vi "Basic Set Address.vi"(6 "chip select  (1st chip)":enum16{"1st chip", "2nd chip"}(ring), 7 "address type (DDRAM)":enum16{"DDRAM", "CGRAM"}(ring), 8 "error in (no error)":errorcluster, 9 "address (0, 0)":u8 format="%.0x", 11 "cluster of private data in":T1={"FPGA VI Reference"=refnum, "device index"=0, "screen size"=enum."8x1", "font size"=enum."5x8", "auto wrap"=FALSE, "alignment"=enum."None", "number of line"=enum."2 lines", "shift 0"=0, "entry mode 0"=enum."increment & no shift", "shift 1"=0, "entry mode 1"=enum."increment & no shift"}) -> (0 "error out":errorcluster, 3 "cluster of private data out":T1={"FPGA VI Reference"=refnum, "device index"=0, "screen size"=enum."8x1", "font size"=enum."5x8", "auto wrap"=FALSE, "alignment"=enum."None", "number of line"=enum."2 lines", "shift 0"=0, "entry mode 0"=enum."increment & no shift", "shift 1"=0, "entry mode 1"=enum."increment & no shift"})   [LabVIEW 2017, in "HD44780.lvclass"]
uses:
  HD44780.lvclass
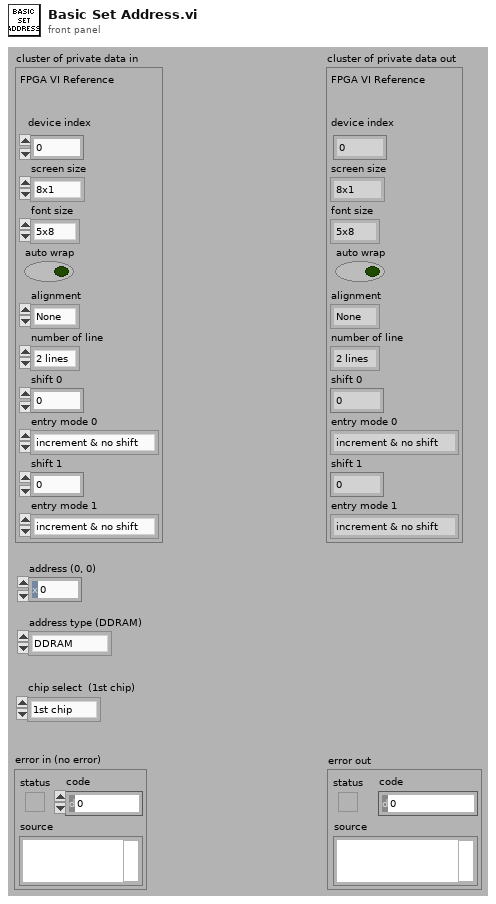
[diagram p1: front panel]
types:
  T1 = cluster{"FPGA VI Reference":refnum<k20>, "device index":i8, "screen size":enum8{"8x1", "8x2", "12x4", "16x1", "16x2", "16x4", "20x1", "20x2", "20x4", "24x1", "24x2", "40x2", "40x4"}, "font size":enum8{"5x8", "5x10"}, "auto wrap":bool, "alignment":enum16{"None", "Left", "Center", "Right"}, "number of line":enum8{"1 line", "2 lines"}, "shift 0":i8, "entry mode 0":enum8{"increment & no shift", "increment & shift", "decrement & no shift", "decrement & shift"}, "shift 1":i8, "entry mode 1":enum8{"increment & no shift", "increment & shift", "decrement & no shift", "decrement & shift"}}
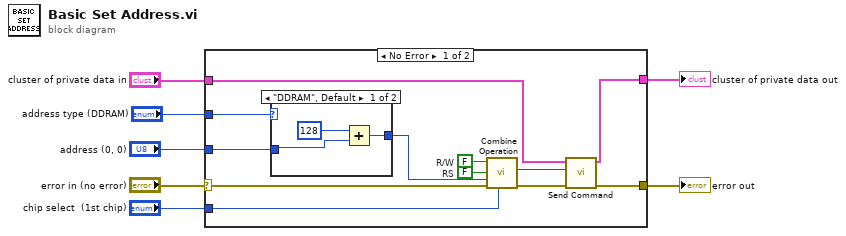
[diagram p0: block diagram]
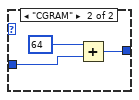
[diagram p2: hidden frame]
diagram:
  n1 = case shown="No Error" "error in (no error)" {
    selector: "error in (no error)" -> [w9 w27]
    tunnel: [w16 w27] -> w7
    tunnel: "cluster of private data in" -> [w8 w26]
    tunnel: "chip select  (1st chip)" -> [w10 _]
    tunnel: "address type (DDRAM)" -> [w13 _]
    tunnel: "address (0, 0)" -> [w12 _]
    tunnel: [w11 w26] -> w1
    frame No Error {
      w14 = FALSE  # RS
      w19 = FALSE  # R/W
      n2 = case shown="\"DDRAM\", Default" w13 {
        tunnel: w12 -> [w21 w25]
        tunnel: [w20 w23] -> w18
        frame "DDRAM", Default {
          n3 = Add(x=u8 128, y=w21) -> (x+y=w20:u8)
        }
        frame "CGRAM" {
          n4 = Add(x=u8 64, y=w25) -> (x+y=w23:u8)
        }
      }
      n5 = call "Combine Operation.vi"("chip select  (1st chip)"=w10, "error in (no error)"=w9, "cmd/data"=w18, "RS"=w14, "R/W"=w19) -> ("error out"=w17:errorcluster, "output"=w15:u32)  [unwired: 5 in]
      n6 = call "Send Command.vi"("error in (no error)"=w17, "operation"=w15, "cluster of private data in"=w8) -> ("error out"=w16:errorcluster, "cluster of private data out"=w11:T1)  [unwired: 6 in, 1 out]
    }
    frame Error {
    }
  }
  "error out" <- w7
  "cluster of private data out" <- w1
